vi "TransmitData.vi"(8 "error in (no error)":errorcluster, 10 "Def-TransmitData":T1, 11 "CAN-NI in":refnum<class "CAN-NI.lvclass">) -> (0 "error out":errorcluster, 3 "CAN-NI out":refnum<class "CAN-NI.lvclass">)   [LabVIEW 2019, in "CAN-NI.lvlib" / "CAN-NI.lvclass"]
uses:
  CAN-NI.lvclass
  CAN-Interface/TypeDef/Def-TransmitData.ctl
  CAN-Interface/TypeDef/Def-PayLoad.ctl
  <vilib>/xnet/xnet.llb/XNET Frame CAN.ctl
  <vilib>/xnet/xnet.llb/XNET Frame Type CAN.ctl
  <vilib>/xnet/xnet.llb/XNET Write (Frame CAN).vi
  CAN-Interface/Class-Interface.lvclass
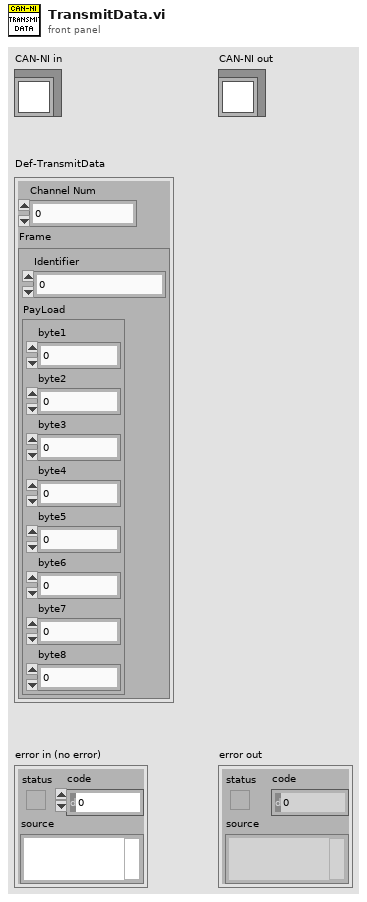
[diagram p1: front panel]
types:
  T1 = typedef "CAN-Interface.lvlib/Class-Interface.lvclass/Def-TransmitData.ctl" = cluster{"Channel Num":u32, "Frame":cluster{"Identifier":u32, "PayLoad":T2}}
  T2 = typedef "CAN-Interface.lvlib/Class-Interface.lvclass/Def-PayLoad.ctl" = cluster{"byte1":u8, "byte2":u8, "byte3":u8, "byte4":u8, "byte5":u8, "byte6":u8, "byte7":u8, "byte8":u8}
  T3 = typedef "XNET Frame CAN.ctl" = cluster{"timestamp":timestamp, "payload":u8[], "identifier":u32, "type":T4, "extended?":bool, "echo?":bool}
  T4 = typedef "XNET Frame Type CAN.ctl" = u8
  T5 = typedef "CAN-NI.lvlib/CAN-NI.lvclass/ChannelProperty.ctl" = cluster{"CAN-cluster":refnum<k21>, "CAN-Frames":refnum<k21>[], "Termination":T6, "Transmit Mode":T7, "Frame Out Session":refnum<k21>, "Frame In Session":refnum<k21>, "Protocol":T8}
  T6 = typedef "CAN-Interface.lvlib/Class-Interface.lvclass/Def-Termination.ctl" = enum8{"on", "off"}
  T7 = typedef "CAN-Interface.lvlib/Class-Interface.lvclass/Def-Transmit Mode.ctl" = enum16{"Queued", "Stream"}
  T8 = typedef "CAN-Interface.lvlib/Class-Interface.lvclass/Def-Protocol.ctl" = enum16{"CAN", "CAN FD"}
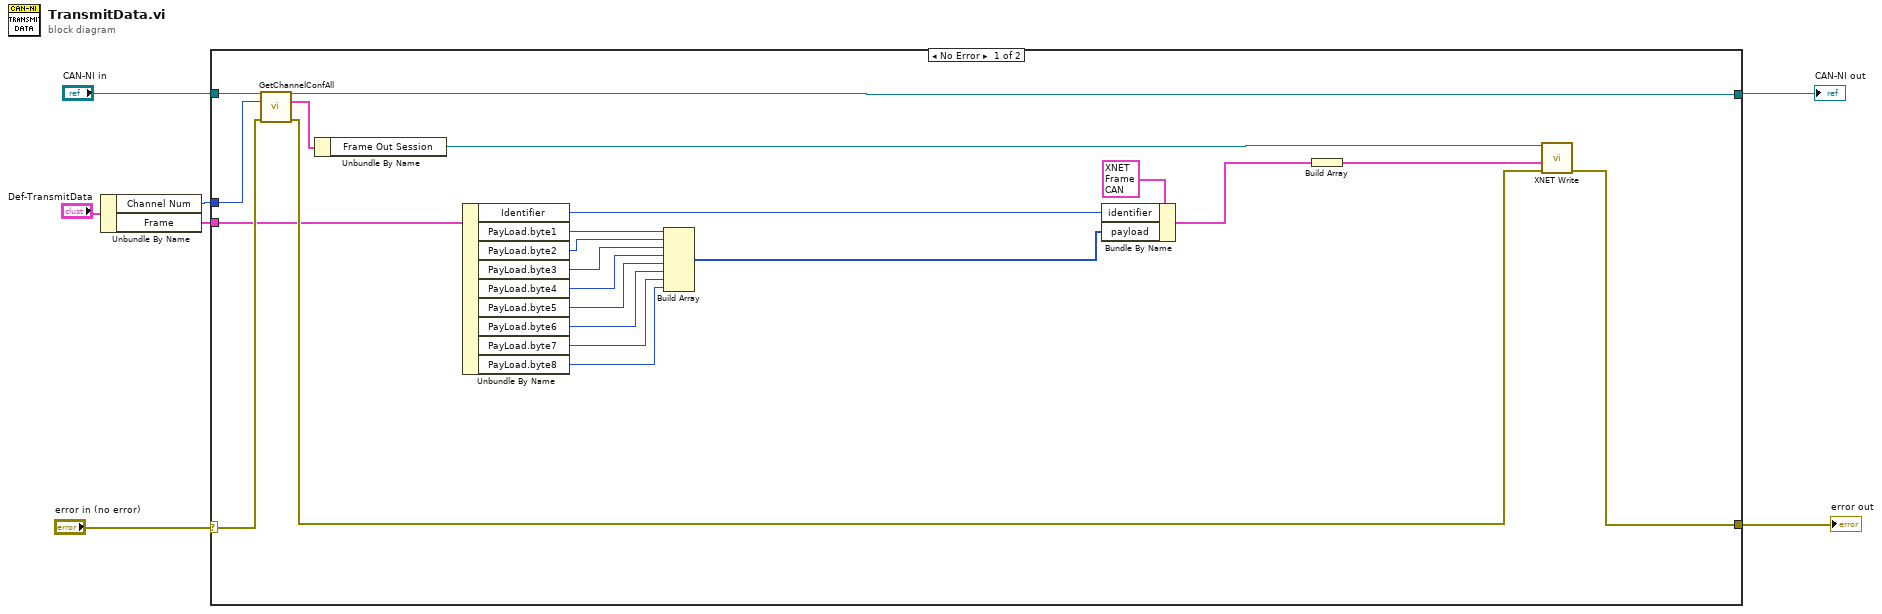
[diagram p0: block diagram]
diagram:
  n1 = Unbundle By Name("Def-TransmitData") -> ("Channel Num"=w2:u32, "Frame"=w1:cluster{"Identifier":u32, "PayLoad":T2})
  n2 = case shown="No Error" "error in (no error)" {
    selector: "error in (no error)" -> [w27 w30]
    tunnel: "CAN-NI in" -> [w29 w31]
    tunnel: w2 -> [w28 _]
    tunnel: w1 -> [w18 _]
    tunnel: [w22 w30] -> w5
    tunnel: [w21 w31] -> w4
    frame No Error {
      n3 = call "GetChannelConfAll.vi"("error in"=w27, "Channel Num"=w28, "CAN-NI"=w29) -> ("error out"=w23:errorcluster, "ChannelProperty"=w26:T5, "CAN-NI"=w21:refnum<class "CAN-NI.lvclass">)  [unwired: 6 in]
      n4 = Unbundle By Name(w26) -> ("Frame Out Session"=w25:refnum<k21>)
      n5 = Unbundle By Name(w18) -> ("Identifier"=w17:u32, "PayLoad.byte1"=w16:u8, "PayLoad.byte2"=w15:u8, "PayLoad.byte3"=w14:u8, "PayLoad.byte4"=w13:u8, "PayLoad.byte5"=w12:u8, "PayLoad.byte6"=w11:u8, "PayLoad.byte7"=w10:u8, "PayLoad.byte8"=w9:u8)
      n6 = Build Array(w16, w15, w14, w13, w12, w11, w10, w9) -> (w8:u8[])
      n7 = Bundle By Name(cluster=T3 {"timestamp"=timestamp(0 s since 1904-01-01), "payload"=[], "identifier"=0, "type"=0, "extended?"=FALSE, "echo?"=FALSE} ("CAN frame"), "identifier"=w17, "payload"=w8) -> (w24:T3)
      n8 = Build Array(w24) -> (w19:T3[])
      n9 = call-poly <vilib>:"XNET Write.vi"("session in"=w25, "data"=w19, "error in (no error)"=w23) -> ("error out"=w22:errorcluster)  [unwired: 11 in, 1 out]
    }
    frame Error {
    }
  }
  "error out" <- w5
  "CAN-NI out" <- w4
